vi "4Pi 4Pi Modes - Write DM.vi"(0 "DM Handles":T1(array[cluster]), 1 "Error In":errorcluster, 2 "No hardware":bool=TRUE, 3 "Norm Voltage (-1, 1)":dbl[](array[numeric])) -> (6 "Error Out":errorcluster)   [LabVIEW 2016]
uses:
  <userlib>/BMC/BMC.lvlib
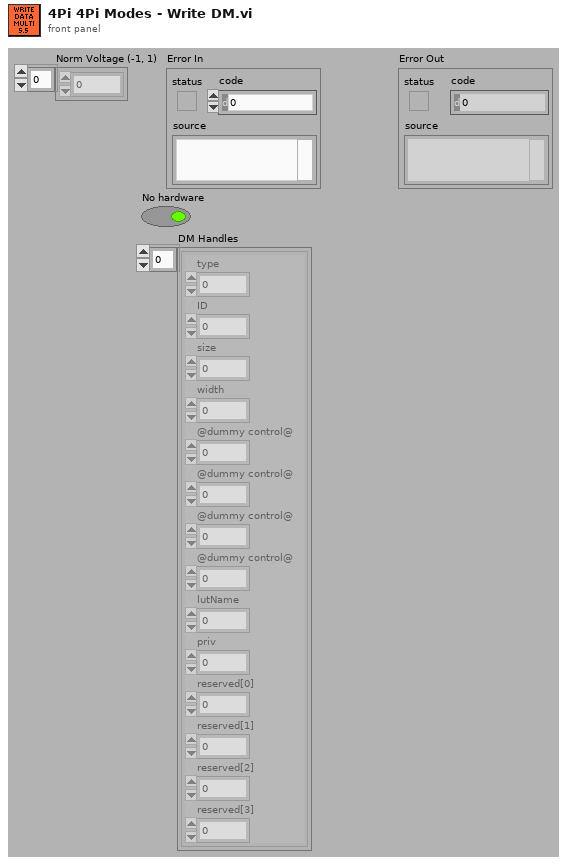
[diagram p1: front panel]
types:
  T1 = cluster{"type":i16, "ID":i16, "size":i32, "width":i32, "@dummy control@":i8, "@dummy control@":i8, "@dummy control@":i8, "@dummy control@":i8, "lutName":u64, "priv":u64, "reserved[0]":i32, "reserved[1]":i32, "reserved[2]":i32, "reserved[3]":i32}[]
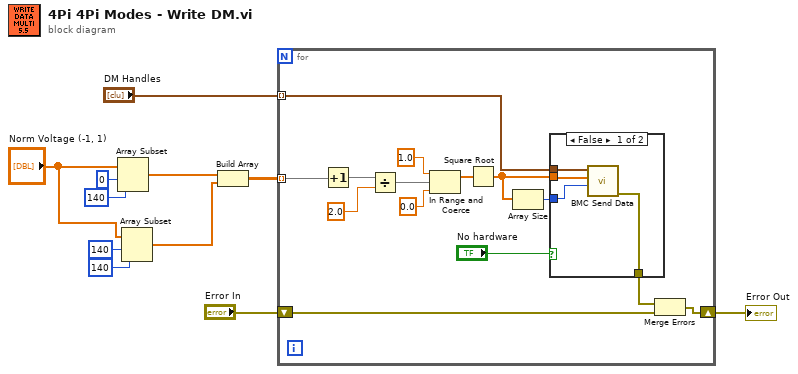
[diagram p0: block diagram]
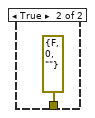
[diagram p2: hidden frame]
diagram:
  n1 = Array Subset(array="Norm Voltage (-1, 1)", index=0, length=140) -> (w6:dbl[])
  n2 = Array Subset(array="Norm Voltage (-1, 1)", index=140, length=140) -> (w5:dbl[])
  n3 = Build Array(w6, w5) -> (w4:dbl[][])
  n4 = for {
    tunnel: w4 -> [w25] mode=indexing
    tunnel: "DM Handles" -> [w19] mode=indexing
    shift-right: [w15] -> w2
    shift-left: "Error In" -> [w16]
    n5 = Increment(x=w25) -> (x+1=w24:dbl[])
    n6 = Divide(x=w24, y=2.0 ("x")) -> (x/y=w22:dbl[])
    n7 = In Range and Coerce(upper limit=1.0 ("x"), x=w22, lower limit=0.0 ("x")) -> (coerced(x)=w14:dbl[])  [unwired: 1 out]
    n8 = Square Root(x=w14) -> (sqrt(x)=w13:dbl[])
    n9 = Array Size(array=w13) -> (size(s)=w18:i32)
    n10 = case shown="False" "No hardware" {
      tunnel: w19 -> [w29 _]
      tunnel: w18 -> [w28 _]
      tunnel: [w27 errorcluster {"status"=FALSE, "code"=0, "source"=""} ("error out")] -> w17
      tunnel: w13 -> [w26 _]
      frame False {
        n11 = call <userlib>:"BMC Send Data.vi"("length"=w28, "data"=w26, "dmHandle"=w29) -> ("error out"=w27:errorcluster)  [unwired: 7 in, 1 out]
      }
      frame True {
      }
    }
    n12 = Merge Errors(w17, w16) -> (w15:errorcluster)
  }
  "Error Out" <- w2
